vi "Ping Actor Msg.vi"(8 "error in (no error)":errorcluster, 10 "Actor":refnum<class "Message Enqueuer.lvclass">) -> (0 "error out":errorcluster, 3 "Ping Actor Msg out":refnum<class "Ping Actor Msg.lvclass">)   [LabVIEW 2020, in "Monitored Actor.lvlib" / "Ping Actor Msg.lvclass"]
uses:
  <vilib>/MGI/Monitored Actor/Actor Monitor/Actor Monitor Messages/Ping Actor Msg/Ping Actor Msg.lvclass
  <vilib>/ActorFramework/Message Enqueuer/Message Enqueuer.lvclass
  <vilib>/MGI/Monitored Actor/Actor Monitor/Actor Monitor Messages/Ping Actor Msg/Ping Actor Msg.lvclass/Ping Actor Msg.ctl
panel:
  in  "Ping Actor Msg in":refnum<class "Ping Actor Msg.lvclass">
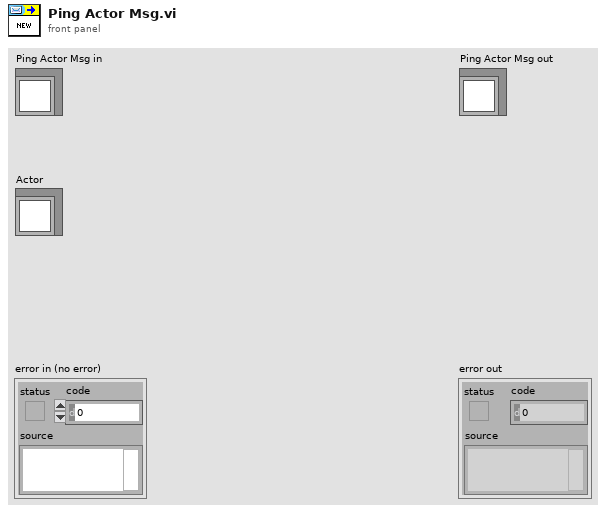
[diagram p1: front panel]
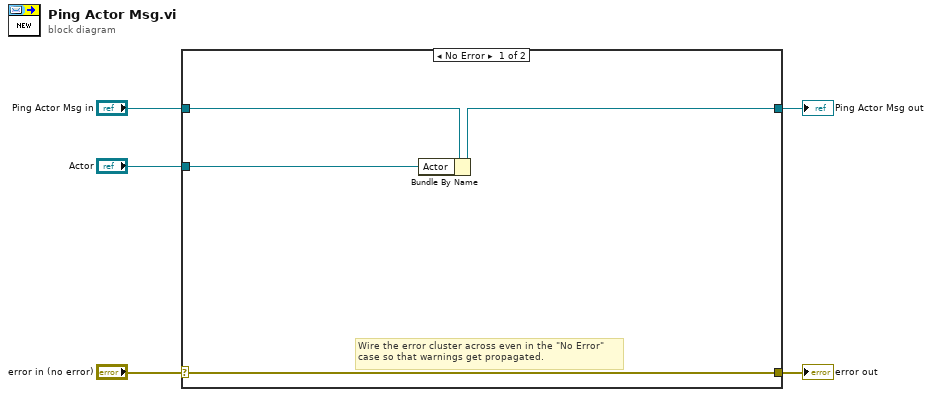
[diagram p0: block diagram]
diagram:
  n1 = case shown="No Error" "error in (no error)" {
    selector: "error in (no error)" -> [w8 w11]
    tunnel: [w8 w11] -> w4
    tunnel: [w7 w10] -> w2
    tunnel: "Ping Actor Msg in" -> [w9 w10]
    tunnel: "Actor" -> [w6 _]
    frame No Error {
      # "Wire the error cluster across even in the \"No Error\"\ncase so that warnings get propagated."
      n2 = Bundle By Name(cluster=w9, "Actor"=w6) -> (w7:refnum<class "Ping Actor Msg.lvclass">)
    }
    frame Error {
    }
  }
  "error out" <- w4
  "Ping Actor Msg out" <- w2
